vi "Close.vi"(8 "error in (no error)":errorcluster, 11 "Measurements in":refnum<class "Measurement.lvclass">) -> (0 "error out":errorcluster, 3 "Measurements out":refnum<class "Measurement.lvclass">)   [LabVIEW 2020, in "Measurement.lvclass"]
uses:
  Measurement.lvclass
  Measurement.lvclass/Measurement.ctl
  Devices/Device.lvclass
  Instruments/Power Supply/Power Supply.lvclass
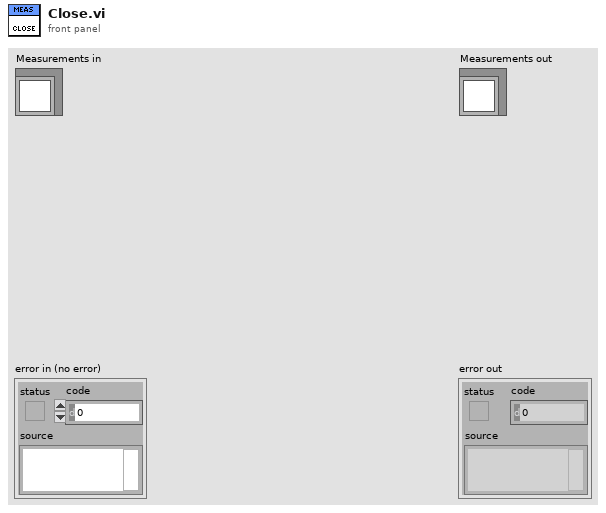
[diagram p1: front panel]
types:
  T1 = typedef "Device.lvclass/DC Offset Cluster.ctl" = cluster{"Enable":bool, "Use Array":bool, "Array":dbl[], "To From Cluster":cluster{"From":dbl, "To":dbl, "Step":dbl}, "Current Value":dbl, "DC Offset":refnum<class "Power Supply.lvclass">}
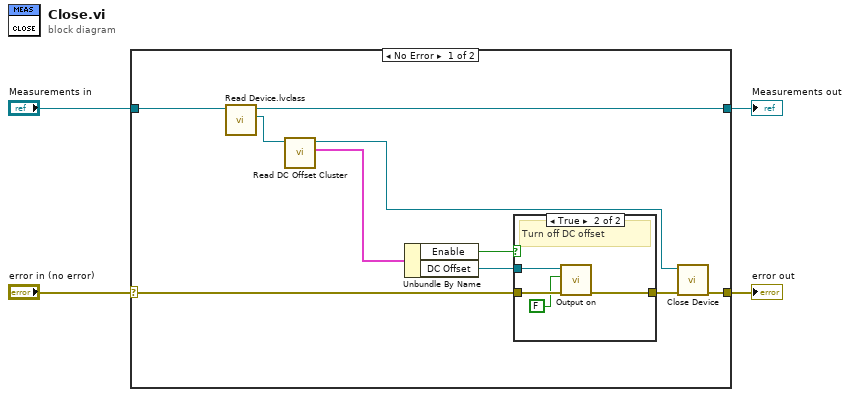
[diagram p0: block diagram]
diagram:
  n1 = case shown="No Error" "error in (no error)" {
    selector: "error in (no error)" -> [w10 w21]
    tunnel: [w5 w21] -> w3
    tunnel: [w8 w20] -> w1
    tunnel: "Measurements in" -> [w9 w20]
    frame No Error {
      n2 = call "Read Device.lvclass.vi"("Measurements in"=w9) -> ("Device.lvclass"=w11:refnum<class "Device.lvclass">, "Measurements out"=w8:refnum<class "Measurement.lvclass">)  [unwired: 9 in]
      n3 = call-dynamic "Read DC Offset Cluster.vi"("Device in"=w11) -> ("DC Offset Cluster"=w12:T1, "Device out"=w6:refnum<class "Device.lvclass">)  [unwired: 8 in, 1 out]
      n4 = Unbundle By Name(w12) -> ("Enable"=w14:bool, "DC Offset"=w13:refnum<class "Power Supply.lvclass">)
      n5 = case shown="True" w14 {
        tunnel: w10 -> [w15 w19]
        tunnel: w13 -> [_ w18]
        tunnel: [w15 w17] -> w7
        frame False {
        }
        frame True {
          # "Turn off DC offset"
          n6 = call-dynamic "Output on.vi"("error in (no error)"=w19, "Output On"=FALSE, "Power Supply in"=w18) -> ("error out"=w17:errorcluster)  [unwired: 7 in, 1 out]
        }
      }
      n7 = call-dynamic "Close Device.vi"("error in (no error)"=w7, "Device in"=w6) -> ("error out"=w5:errorcluster)  [unwired: 8 in, 1 out]
    }
    frame Error {
    }
  }
  "error out" <- w3
  "Measurements out" <- w1
